vi "MAIN_CREAR_BANDEJA.vi"(8 "error in (no error)":errorcluster) -> (0 "error in (no error) 2":errorcluster, 1 "fichero bandeja selecc":path)   [LabVIEW 2019]
uses:
  Type_defs/Array_deClusterBandeja.ctl
  Type_defs/ESTADOS_CREAR_BANDEJA.ctl
  Type_defs/Refs_controles_input_Bandeja.ctl
panel:
  out "DATOS DE BANDEJA SELECCIONADA":T1
  in  "Tab depuracion":enum32{"Page 1"}(tab)
  out "Array Clusters Bandejas":T2
  out "FICHEROS .DB EN CARPETA BANDEJAS":string[](array[string])
  out "ESTADO ACTUAL":T3
  in  "Tab Control":enum32{"Page 1", "Page 2"}(tab)
  in  "Cancel":bool
  in  "CREAR BANDEJA NUEVA":bool
  in  "SELECCIONAR BANDEJA":bool
  in  "GUARDAR BANDEJA":bool
  in  "largo (mm)":u32
  in  "Paso X (mm)":dbl
  in  "ancho (mm)":u32
  in  "Paso Y (mm)":dbl
  in  "DISTANCIA SUELO bANDEJA A CHIP (mm)":dbl
  in  "Nº de filas":u32
  in  "Nº de columnas":u32
  in  "Dist. borde bandeja a centro chip (mm)":dbl
  in  "nombre bandeja":string
  in  "SELECTOR BANDEJA":string(combo)
  out "RUTA CARPETA BANDEJAS":path
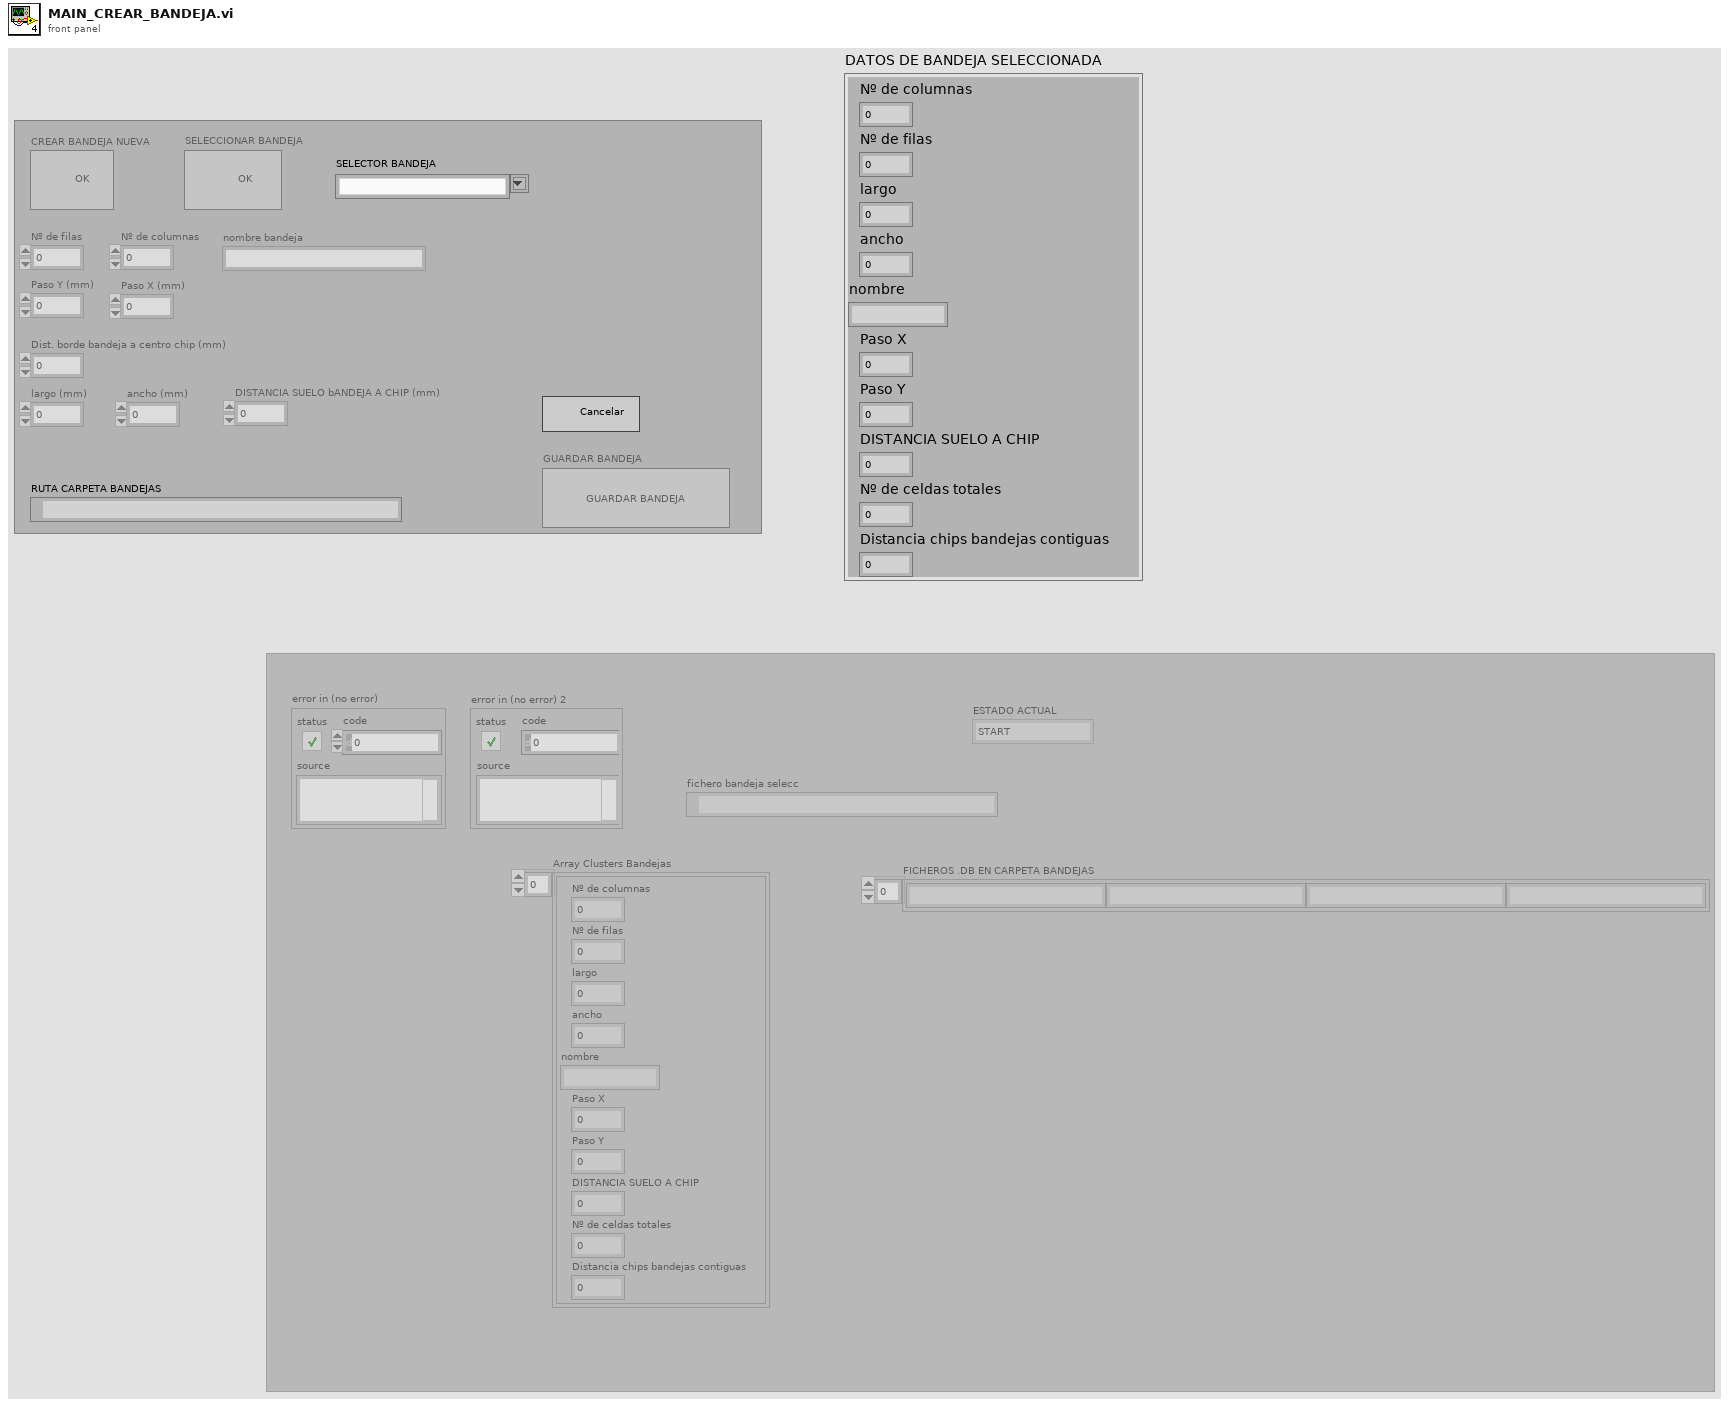
[diagram p1: front panel]
types:
  T1 = cluster{"Nº de columnas ":u32, "Nº de filas ":u32, "largo":u32, "ancho":u32, "nombre":string, "Paso X":dbl, "Paso Y":dbl, "DISTANCIA SUELO A CHIP  ":dbl, "Nº de celdas totales":u16, "Distancia chips bandejas contiguas":dbl}
  T2 = typedef "Array_deClusterBandeja.ctl" = cluster{"Nº de columnas ":u32, "Nº de filas ":u32, "largo":u32, "ancho":u32, "nombre":string, "Paso X":dbl, "Paso Y":dbl, "DISTANCIA SUELO A CHIP  ":dbl, "Nº de celdas totales":u16, "Distancia chips bandejas contiguas":dbl}[]
  T3 = typedef "ESTADOS_CREAR_BANDEJA.ctl" = enum16{"START", "PROMPT MESSAGE", "BANDEJA NUEVA?", "FLAG_BANDEJA_NUEVA", "GUARDAR BANDEJA NUEVA", "GESTION EVENTOS", "LEER BANDEJAS", "OTRA BANDEJA?", "ACTUALIZAR SELECTOR", "ERROR?", "SALIR"}
  T4 = typedef "Refs_controles_input_Bandeja.ctl" = cluster{"NºFILAS":refnum<vi>, "NºCOLUMNAS":refnum<vi>, "DISTANCIA SUELO CHIP":refnum<vi>, "PASOX":refnum<vi>, "PASOY":refnum<vi>, "ANCHO":refnum<vi>, "LARGO":refnum<vi>, "DIST.BORDE BANDEJA A CHIP":refnum<vi>, "NOMBRE BANDEJA":refnum<vi>}
  T5 = enum8{"Enabled", "Disabled", "Disabled and Grayed Out"}
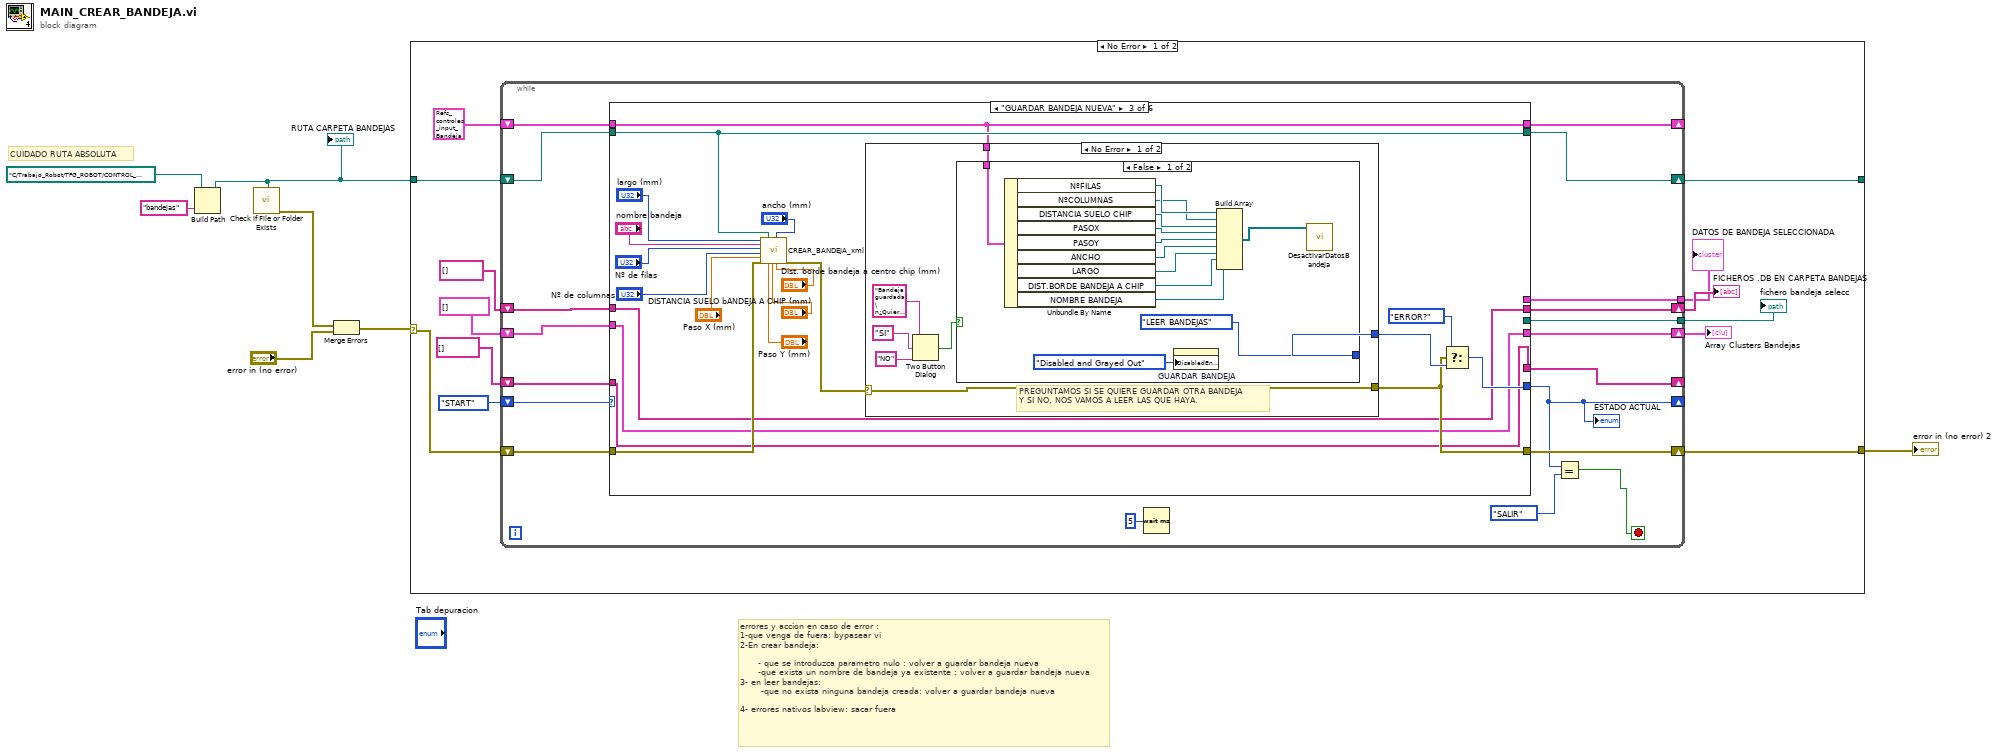
[diagram p0: block diagram]
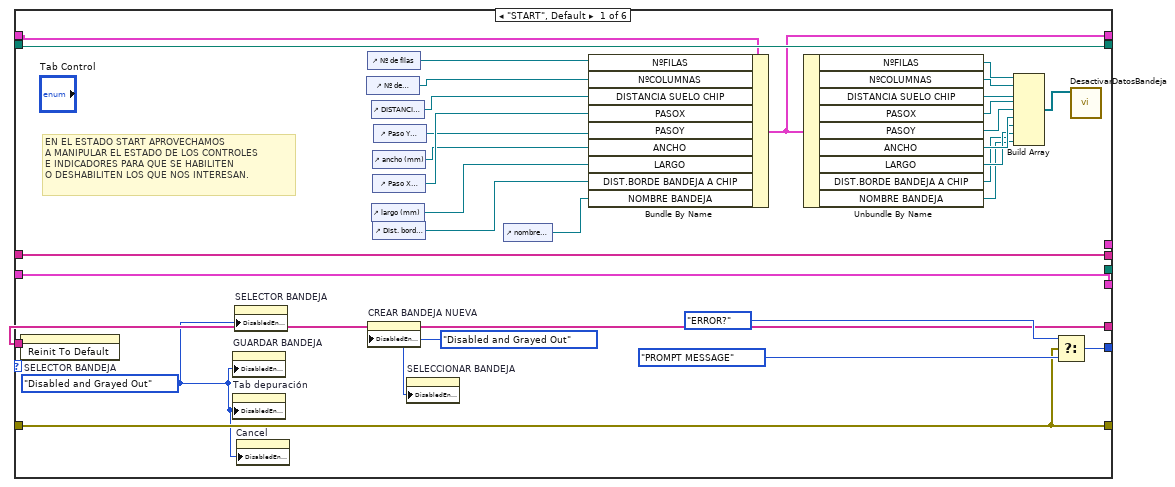
[diagram p2: hidden frame]
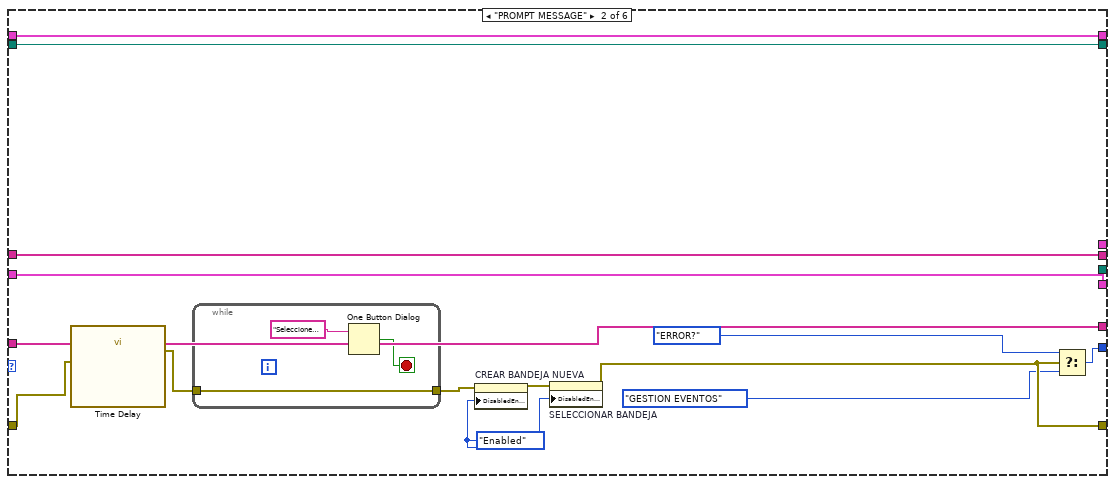
[diagram p3: hidden frame]
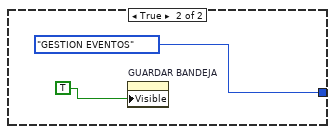
[diagram p4: hidden frame]
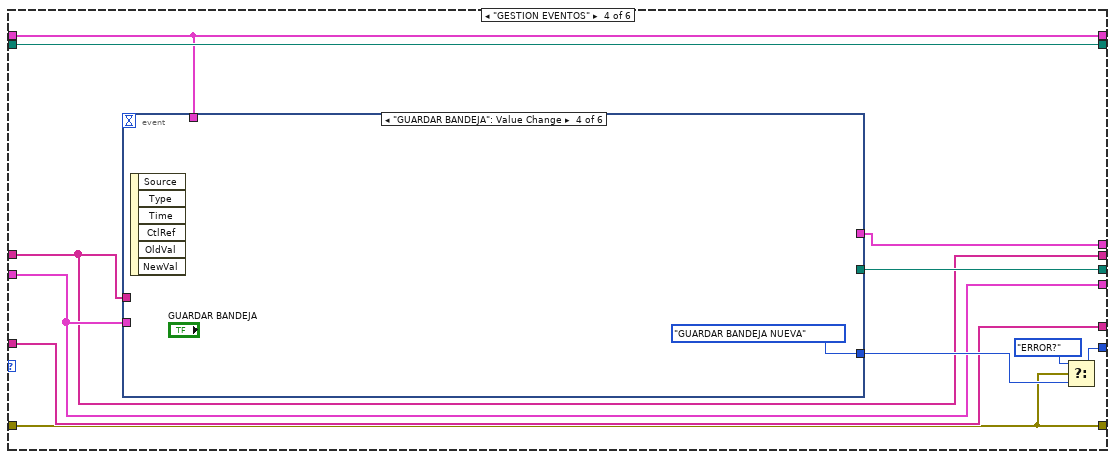
[diagram p6: hidden frame]
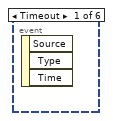
[diagram p7: hidden frame]
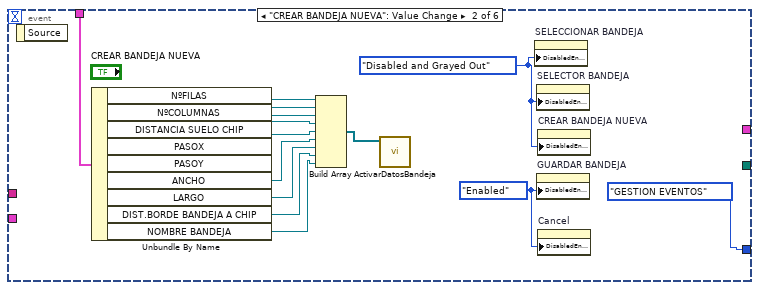
[diagram p8: hidden frame]
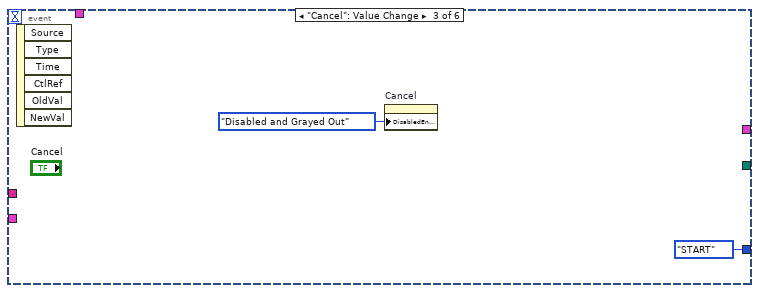
[diagram p9: hidden frame]
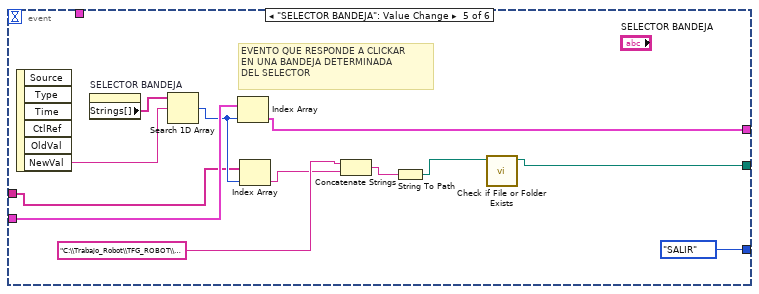
[diagram p10: hidden frame]
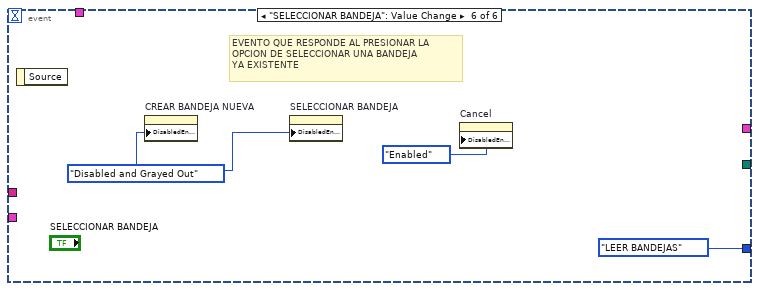
[diagram p11: hidden frame]
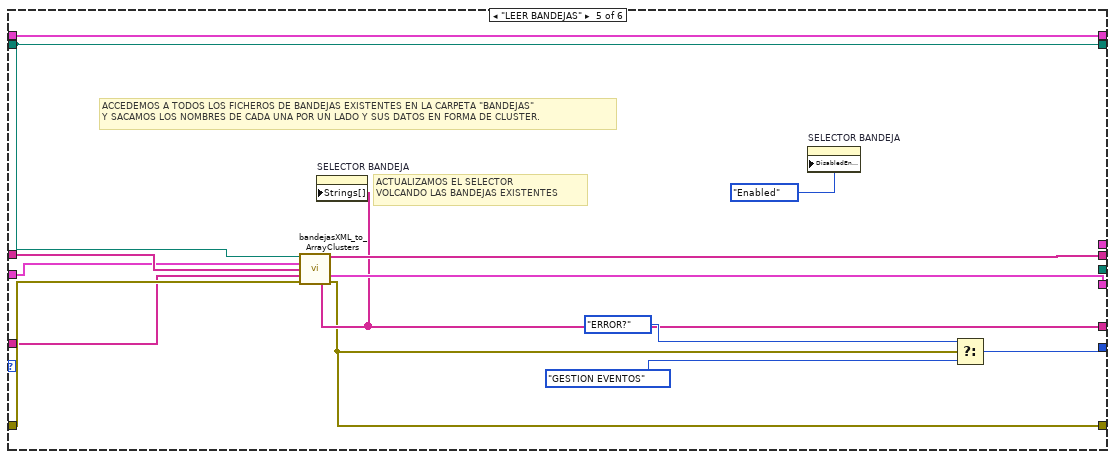
[diagram p12: hidden frame]
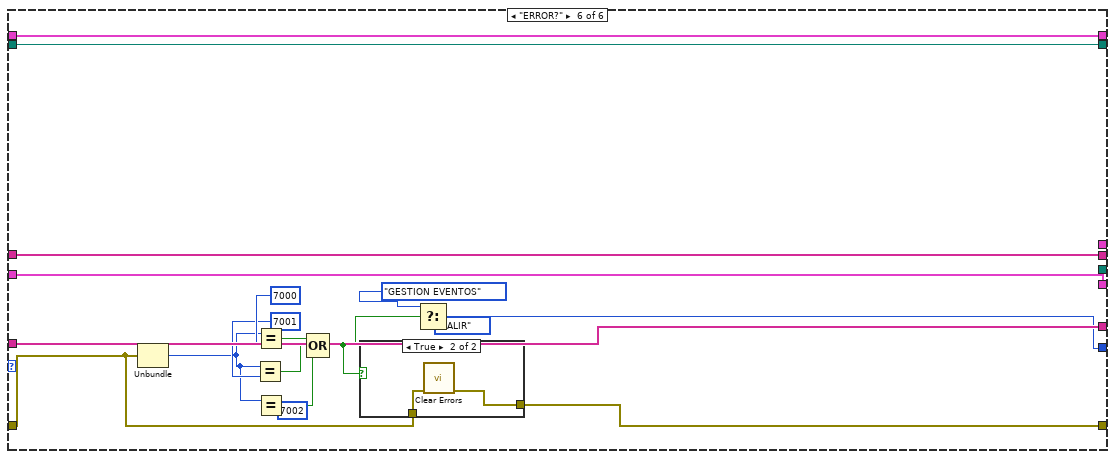
[diagram p13: hidden frame]
diagram:
  # "CUIDADO RUTA ABSOLUTA"
  # "errores y accion en caso de error :\n1-que venga de fuera: bypasear vi\n2-En crear bandeja:\n\n      - que se introduzca parametro nulo : volver a guardar bandeja nueva\n      -que exista un nombre de bandeja ya existente : volver a guardar bandeja nueva\n3- en leer bandejas:\n       -que no exista ninguna bandeja creada: volver a guardar bandeja nueva\n\n4- errores nativos labview: sacar fuera"
  n1 = Build Path(base path=path "C:/Trabajo_Robot/TFG_ROBOT/CONTROL_ROBOT", name or relative path="bandejas") -> (appended path=w5:path)
  "RUTA CARPETA BANDEJAS" <- w5
  n2 = call <vilib>:"Check if File or Folder Exists.vi"("path"=w5) -> ("error out"=w2:errorcluster)  [unwired: 8 in, 2 out]
  n3 = Merge Errors(w2, "error in (no error)") -> (w4:errorcluster)
  n4 = case shown="No Error" w4 {
    selector: w4 -> [w15 w210]
    tunnel: [w17 w210] -> w6
    tunnel: w5 -> [w16 w209]
    tunnel: [w10 w209] -> _
    frame No Error {
      n5 = while {
        shift-right: [w37] -> w17
        shift-left: w15 -> [w38]
        shift-right: [w23] -> _
        shift-left: ESTADOS_CREAR_BANDEJA."START" ("Enum") -> [w39]
        shift-right: [w35] -> w10
        shift-left: w16 -> [w36]
        shift-right: [w34] -> _
        shift-left: string[] [] ("Nombres bandejas") -> [w31]
        shift-right: [w33] -> w13
        shift-left: string[] [] ("filenames") -> [w30]
        shift-right: [w32] -> w12
        shift-left: T2 [] ("Array Clusters Bandejas") -> [w29]
        tunnel: [w28] -> w8
        shift-right: [w24] -> _
        shift-left: T4 {"NºFILAS"=refnum, "NºCOLUMNAS"=refnum, "DISTANCIA SUELO CHIP"=refnum, "PASOX"=refnum, "PASOY"=refnum, "ANCHO"=refnum, "LARGO"=refnum, "DIST.BORDE BANDEJA A CHIP"=refnum, "NOMBRE BANDEJA"=refnum} ("Refs. controles datos bandeja") -> [w25]
        tunnel: [w21] -> w9
        stop <- w22 stop-if-true
        n6 = case shown="\"GUARDAR BANDEJA NUEVA\"" w39 {
          tunnel: w38 -> [w41 w72 w95 w134 w185 w192]
          tunnel: [w41 w76 w93 w134 w177 w193] -> w37
          tunnel: [w68 w84 w96 w140 w182 w189] -> w23
          tunnel: w36 -> [w67 w80 w89 w138 w176 w202]
          tunnel: [w67 w80 w89 w138 w176 w202] -> w35
          tunnel: [w66 w83 w92 w137 w181 w205] -> w34
          tunnel: [w65 w82 w90 w132 w187 w204] -> w33
          tunnel: [w64 w81 w91 w136 w186 w203] -> w32
          tunnel: w31 -> [w66 w83 w92 w137 w180 w205]
          tunnel: w30 -> [w65 w82 w90 w132 w179 w204]
          tunnel: w29 -> [w64 w81 w91 w136 w178 w203]
          tunnel: [_ _ _ w131 _ _] -> w28
          tunnel: w25 -> [w43 w73 w88 w135 w174 w188]
          tunnel: [w42 w73 w88 w135 w174 w188] -> w24
          tunnel: [_ _ _ w133 _ _] -> w21
          frame "START", Default {
            w63 = T5."Disabled and Grayed Out" ("Disabled")
            w40 = T5."Disabled and Grayed Out" ("Disabled")
            # "EN EL ESTADO START APROVECHAMOS\nA MANIPULAR EL ESTADO DE LOS CONTROLES\nE INDICADORES PARA QUE SE HABILITEN\nO DESHABILITEN LOS QUE NOS INTERESAN."
            n7 = invoke on="SELECTOR BANDEJA" class="CmbBox" method="Reinit To Default"() -> ()  [unwired: 3 in, 3 out]
            n8 = property on="GUARDAR BANDEJA" class="Bool"("DisabledEnum"=w40) -> ()  [unwired: 2 in, 2 out]
            n9 = property on="Tab depuración" class="TabCtl (strict)"("DisabledEnum"=w40) -> ()  [unwired: 2 in, 2 out]
            n10 = property on="SELECTOR BANDEJA" class="CmbBox"("DisabledEnum"=w40) -> ()  [unwired: 2 in, 2 out]
            n11 = property on="Cancel" class="Bool"("DisabledEnum"=w40) -> ()  [unwired: 2 in, 2 out]
            n12 = control-ref of="Nº de columnas"() -> (w61:refnum<vi>)
            n13 = control-ref of="Nº de filas"() -> (w62:refnum<vi>)
            n14 = property on="CREAR BANDEJA NUEVA" class="Bool"("DisabledEnum"=w63) -> ()  [unwired: 2 in, 2 out]
            n15 = control-ref of="DISTANCIA SUELO bANDEJA A CHIP (mm)"() -> (w60:refnum<vi>)
            n16 = control-ref of="largo (mm)"() -> (w56:refnum<vi>)
            n17 = control-ref of="ancho (mm)"() -> (w57:refnum<vi>)
            n18 = control-ref of="Paso X (mm)"() -> (w59:refnum<vi>)
            n19 = control-ref of="Dist. borde bandeja a centro chip (mm)"() -> (w55:refnum<vi>)
            n20 = control-ref of="Paso Y (mm)"() -> (w58:refnum<vi>)
            n21 = property on="SELECCIONAR BANDEJA" class="Bool"("DisabledEnum"=w63) -> ()  [unwired: 2 in, 2 out]
            n22 = control-ref of="nombre bandeja"() -> (w54:refnum<vi>)
            n23 = Bundle By Name(cluster=w43, "NºFILAS"=w62, "NºCOLUMNAS"=w61, "DISTANCIA SUELO CHIP"=w60, "PASOX"=w59, "PASOY"=w58, "ANCHO"=w57, "LARGO"=w56, "DIST.BORDE BANDEJA A CHIP"=w55, "NOMBRE BANDEJA"=w54) -> (w42:T4)
            n24 = Unbundle By Name(w42) -> ("NºFILAS"=w53:refnum<vi>, "NºCOLUMNAS"=w52:refnum<vi>, "DISTANCIA SUELO CHIP"=w51:refnum<vi>, "PASOX"=w50:refnum<vi>, "PASOY"=w49:refnum<vi>, "ANCHO"=w48:refnum<vi>, "LARGO"=w47:refnum<vi>, "DIST.BORDE BANDEJA A CHIP"=w46:refnum<vi>, "NOMBRE BANDEJA"=w45:refnum<vi>)
            n25 = Build Array(w53, w52, w51, w50, w49, w48, w47, w46, w45) -> (w44:refnum<vi>[])
            n26 = Select(t=ESTADOS_CREAR_BANDEJA."ERROR?", s=w41, f=ESTADOS_CREAR_BANDEJA."PROMPT MESSAGE") -> (s? t:f=w68:T3)
            n27 = call "DesactivarDatosBandeja.vi"("Array"=w44) -> ()  [unwired: 11 in]
          }
          frame "PROMPT MESSAGE" {
            w79 = T5."Enabled" ("Disabled")
            n28 = call "Time Delay"("error in (no error)"=w72) -> ("error out"=w71:errorcluster)  [unwired: 10 in]
            n29 = while {
              tunnel: w71 -> [w85]
              tunnel: [w85] -> w78
              stop <- w86 stop-if-true
              n30 = One Button Dialog(message="Seleccione tipo de bandeja o pulse crear una nueva") -> (true=w86:bool)  [unwired: 1 in]
            }
            n31 = property on="CREAR BANDEJA NUEVA" class="Bool"(error in=w78, "DisabledEnum"=w79) -> (error out=w77:errorcluster)  [unwired: 1 in, 1 out]
            n32 = property on="SELECCIONAR BANDEJA" class="Bool"(error in=w77, "DisabledEnum"=w79) -> (error out=w76:errorcluster)  [unwired: 1 in, 1 out]
            n33 = Select(t=ESTADOS_CREAR_BANDEJA."ERROR?" ("f"), s=w76, f=ESTADOS_CREAR_BANDEJA."GESTION EVENTOS" ("Enum")) -> (s? t:f=w84:T3)
          }
          frame "GUARDAR BANDEJA NUEVA" {
            n34 = call "CREAR_BANDEJA_xml.vi"("largo"="largo (mm)", "nombre bandeja"="nombre bandeja", "Nº de filas"="Nº de filas", "Nº de columnas"="Nº de columnas", "Paso X"="Paso X (mm)", "error in (no error)"=w95, "path"=w89, "Paso Y"="Paso Y (mm)", "DISTANCIA SUELO A CHIP"="DISTANCIA SUELO bANDEJA A CHIP (mm)", "ancho"="ancho (mm)", "Dist. borde bandeja a centro chip"="Dist. borde bandeja a centro chip (mm)") -> ("error out"=w94:errorcluster)  [unwired: 8 in]
            n35 = case shown="No Error" w94 {
              selector: w94 -> [w109 w130]
              tunnel: [w110 _] -> w97
              tunnel: [w109 w130] -> w93
              tunnel: w88 -> [w108 _]
              frame No Error {
                # "PREGUNTAMOS SI SE QUIERE GUARDAR OTRA BANDEJA\nY SI NO, NOS VAMOS A LEER LAS QUE HAYA."
                n36 = Two Button Dialog(message="Bandeja guardada!\n¿Quieres crear otra bandeja?", 1:"NO" ("F button name (\"Cancel\")"), 2:"SI" ("T button name (\"OK\")")) -> (T button?=w111:bool)
                n37 = case shown="False" w111 {
                  tunnel: [ESTADOS_CREAR_BANDEJA."LEER BANDEJAS" ESTADOS_CREAR_BANDEJA."GESTION EVENTOS" ("Enum")] -> w110
                  tunnel: w108 -> [w115 _]
                  frame False {
                    n38 = Unbundle By Name(w115) -> ("NºFILAS"=w125:refnum<vi>, "NºCOLUMNAS"=w124:refnum<vi>, "DISTANCIA SUELO CHIP"=w123:refnum<vi>, "PASOX"=w122:refnum<vi>, "PASOY"=w121:refnum<vi>, "ANCHO"=w120:refnum<vi>, "LARGO"=w119:refnum<vi>, "DIST.BORDE BANDEJA A CHIP"=w118:refnum<vi>, "NOMBRE BANDEJA"=w117:refnum<vi>)
                    n39 = property on="GUARDAR BANDEJA" class="Bool"("DisabledEnum"=T5."Disabled and Grayed Out" ("Disabled")) -> ()  [unwired: 2 in, 2 out]
                    n40 = Build Array(w125, w124, w123, w122, w121, w120, w119, w118, w117) -> (w116:refnum<vi>[])
                    n41 = call "DesactivarDatosBandeja.vi"("Array"=w116) -> ()  [unwired: 11 in]
                  }
                  frame True {
                    n42 = property on="GUARDAR BANDEJA" class="Bool"("Visible"=TRUE) -> ()  [unwired: 2 in, 2 out]
                  }
                }
              }
              frame Error {
              }
            }
            n43 = Select(t=ESTADOS_CREAR_BANDEJA."ERROR?", s=w93, f=w97) -> (s? t:f=w96:T3)
          }
          frame "GESTION EVENTOS" {
            n44 = event shown="[3] \"GUARDAR BANDEJA\": Value Change" {
              selector: _ -> [_ _ _ _ _ _]
              dyn-events: _ -> [_ _ _ _ _ _]
              timeout: _ -> [_ _ _ _ _ _]
              tunnel: [_ ESTADOS_CREAR_BANDEJA."GESTION EVENTOS" ("f") ESTADOS_CREAR_BANDEJA."START" ("f") ESTADOS_CREAR_BANDEJA."GUARDAR BANDEJA NUEVA" ("f") ESTADOS_CREAR_BANDEJA."SALIR" ("f") ESTADOS_CREAR_BANDEJA."LEER BANDEJAS" ("f")] -> w139
              tunnel: w136 -> [_ _ _ _ w169 _]
              tunnel: w135 -> [_ w153 _ _ _ _]
              tunnel: w132 -> [_ _ _ _ w165 _]
              tunnel: [_ _ _ _ w160 _] -> w133
              tunnel: [_ _ _ _ w159 _] -> w131
              event Timeout {
                n45 = event-data() -> ()  [unwired: 1 in, 3 out]
              }
              event "CREAR BANDEJA NUEVA": Value Change {
                w142 = T5."Enabled" ("Disabled")
                w154 = T5."Disabled and Grayed Out" ("Disabled")
                n46 = event-data() -> ()  [unwired: 1 in, 1 out]
                n47 = Unbundle By Name(w153) -> ("NºFILAS"=w152:refnum<vi>, "NºCOLUMNAS"=w151:refnum<vi>, "DISTANCIA SUELO CHIP"=w150:refnum<vi>, "PASOX"=w149:refnum<vi>, "PASOY"=w148:refnum<vi>, "ANCHO"=w147:refnum<vi>, "LARGO"=w146:refnum<vi>, "DIST.BORDE BANDEJA A CHIP"=w145:refnum<vi>, "NOMBRE BANDEJA"=w144:refnum<vi>)
                n48 = Build Array(w152, w151, w150, w149, w148, w147, w146, w145, w144) -> (w143:refnum<vi>[])
                n49 = call "ActivarDatosBandeja.vi"("Array"=w143) -> ()  [unwired: 11 in]
                n50 = property on="SELECCIONAR BANDEJA" class="Bool"("DisabledEnum"=w154) -> ()  [unwired: 2 in, 2 out]
                n51 = property on="SELECTOR BANDEJA" class="CmbBox"("DisabledEnum"=w154) -> ()  [unwired: 2 in, 2 out]
                n52 = property on="GUARDAR BANDEJA" class="Bool"("DisabledEnum"=w142) -> ()  [unwired: 2 in, 2 out]
                n53 = property on="CREAR BANDEJA NUEVA" class="Bool"("DisabledEnum"=w154) -> ()  [unwired: 2 in, 2 out]
                n54 = property on="Cancel" class="Bool"("DisabledEnum"=w142) -> ()  [unwired: 2 in, 2 out]
              }
              event "Cancel": Value Change {
                n55 = event-data() -> ()  [unwired: 1 in, 6 out]
                n56 = property on="Cancel" class="Bool"("DisabledEnum"=T5."Disabled and Grayed Out" ("Disabled")) -> ()  [unwired: 2 in, 2 out]
              }
              event "GUARDAR BANDEJA": Value Change {
                n57 = event-data() -> ()  [unwired: 1 in, 6 out]
              }
              event "SELECTOR BANDEJA": Value Change {
                # "EVENTO QUE RESPONDE A CLICKAR\nEN UNA BANDEJA DETERMINADA\nDEL SELECTOR"
                n58 = event-data() -> ("NewVal"=w167:string)  [unwired: 1 in, 5 out]
                n59 = property on="SELECTOR BANDEJA" class="CmbBox"() -> ("Strings[]"=w170:string[])  [unwired: 2 in, 2 out]
                n60 = Search 1D Array(1D array=w170, element=w167) -> (index of element=w166:i32)  [unwired: 1 in]
                n61 = Index Array(array=w169, index=w166) -> (element=w159:T1)
                n62 = Index Array(array=w165, index=w166) -> (element=w163:string)
                n63 = Concatenate Strings("C:\\Trabajo_Robot\\TFG_ROBOT\\CONTROL_ROBOT\\bandejas\\", w163) -> (w162:string)
                n64 = String To Path(string=w162) -> (path=w161:path)
                n65 = call <vilib>:"Check if File or Folder Exists.vi"("path"=w161) -> ("dup path"=w160:path)  [unwired: 8 in, 2 out]
              }
              event "SELECCIONAR BANDEJA": Value Change {
                w172 = T5."Disabled and Grayed Out" ("Disabled")
                # "EVENTO QUE RESPONDE AL PRESIONAR LA\nOPCION DE SELECCIONAR UNA BANDEJA\nYA EXISTENTE"
                n66 = event-data() -> ()  [unwired: 1 in, 1 out]
                n67 = property on="CREAR BANDEJA NUEVA" class="Bool"("DisabledEnum"=w172) -> ()  [unwired: 2 in, 2 out]
                n68 = property on="SELECCIONAR BANDEJA" class="Bool"("DisabledEnum"=w172) -> ()  [unwired: 2 in, 2 out]
                n69 = property on="Cancel" class="Bool"("DisabledEnum"=T5."Enabled" ("Disabled")) -> ()  [unwired: 2 in, 2 out]
              }
            }
            n70 = Select(t=ESTADOS_CREAR_BANDEJA."ERROR?", s=w134, f=w139) -> (s? t:f=w140:T3)
          }
          frame "LEER BANDEJAS" {
            # "ACTUALIZAMOS EL SELECTOR\nVOLCANDO LAS BANDEJAS EXISTENTES"
            # "ACCEDEMOS A TODOS LOS FICHEROS DE BANDEJAS EXISTENTES EN LA CARPETA \"BANDEJAS\"\nY SACAMOS LOS NOMBRES DE CADA UNA POR UN LADO Y SUS DATOS EN FORMA DE CLUSTER."
            n71 = call "bandejasXML_to_ArrayClusters.vi"("path"=w176, "Array Clusters Bandejas"=w178, "Filenames"=w179, "Nombres bandejas"=w180, "error in (no error)"=w185) -> ("Nombres bandejas"=w181:string[], "filenames"=w187:string[], "Array Clusters Bandejas"=w186:T2, "error out"=w177:errorcluster)  [unwired: 7 in]
            n72 = property on="SELECTOR BANDEJA" class="CmbBox"("Strings[]"=w181) -> ()  [unwired: 2 in, 2 out]
            n73 = property on="SELECTOR BANDEJA" class="CmbBox"("DisabledEnum"=T5."Enabled" ("Disabled")) -> ()  [unwired: 2 in, 2 out]
            n74 = Select(t=ESTADOS_CREAR_BANDEJA."ERROR?", s=w177, f=ESTADOS_CREAR_BANDEJA."GESTION EVENTOS") -> (s? t:f=w182:T3)
          }
          frame "ERROR?" {
            n75 = Unbundle(w192) -> ("code"=w194:i32)  [unwired: 2 out]
            n76 = Equal?(x=w194, y=7001) -> (x = y?=w197:bool)
            n77 = Equal?(x=w194, y=7000) -> (x = y?=w198:bool)
            n78 = Equal?(x=w194, y=7002) -> (x = y?=w196:bool)
            n79 = Compound Arithmetic op=OR(w198, w197, w196) -> (w195:bool)
            n80 = case shown="True" w195 {
              tunnel: [w206 w208] -> w193
              tunnel: w192 -> [w206 w207]
              frame False {
              }
              frame True {
                n81 = call <vilib>:"Clear Errors.vi"("error in (no error)"=w207) -> ("error out"=w208:errorcluster)  [unwired: 5 in, 1 out]
              }
            }
            n82 = Select(t=ESTADOS_CREAR_BANDEJA."GESTION EVENTOS" ("Enum"), s=w195, f=ESTADOS_CREAR_BANDEJA."SALIR") -> (s? t:f=w189:T3)
          }
        }
        "ESTADO ACTUAL" <- w23
        n83 = Wait (ms)(milliseconds to wait=u32 5) -> ()  [unwired: 1 out]
        n84 = Equal?(x=w23, y=ESTADOS_CREAR_BANDEJA."SALIR") -> (x = y?=w22:bool)
      }
      "FICHEROS .DB EN CARPETA BANDEJAS" <- w13
      "Array Clusters Bandejas" <- w12
      "fichero bandeja selecc" <- w9
      "DATOS DE BANDEJA SELECCIONADA" <- w8
    }
    frame Error {
    }
  }
  "error in (no error) 2" <- w6
